vi "Create Session directory.vi"(8 "error in (no error)":errorcluster, 10 "Identifier 1":string, 11 "appended path":path) -> (0 "error out":errorcluster, 2 "File name base":string, 3 "created path":path)   [LabVIEW 2016]
panel:
  out "date/time string":string
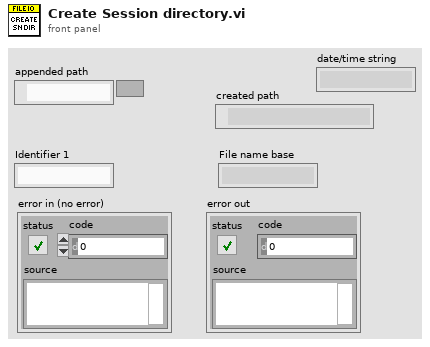
[diagram p1: front panel]
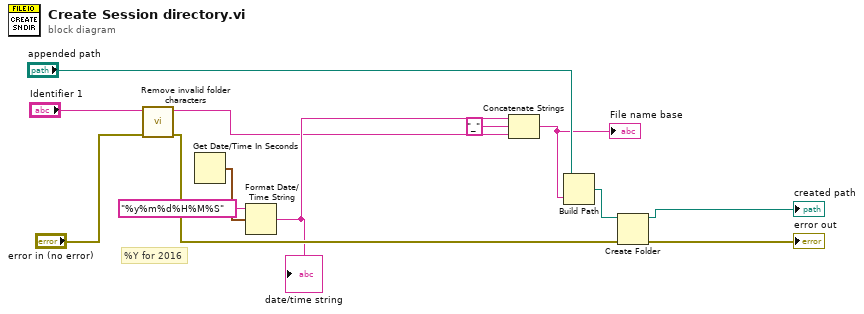
[diagram p0: block diagram]
diagram:
  # "%Y for 2016"
  n1 = call "Remove invalid folder characters.vi"("error in (no error)"="error in (no error)", "String in"="Identifier 1") -> ("error out"=w5:errorcluster, "String out"=w2:string)  [unwired: 8 in]
  n2 = Get Date/Time In Seconds() -> (seconds since 1Jan1904=w7:timestamp)
  n3 = Format Date/Time String(time format string (%c)="%y%m%d%H%M%S", seconds (now)=w7) -> (date/time string=w4:string)  [unwired: 1 in]
  "date/time string" <- w4
  n4 = Concatenate Strings(w4, "_" ("string"), w2) -> (w1:string)
  "File name base" <- w1
  n5 = Build Path(base path="appended path", name or relative path=w1) -> (appended path=w12:path)
  n6 = Create Folder(path (use dialog)=w12, error in=w5) -> (created path=→"created path":path, error out=→"error out":errorcluster)  [unwired: 1 in, 1 out]
